vi "Destroy.vi"   [LabVIEW 2018, in "Toolkit.lvlib" / "Channel.lvclass"]
uses:
  Channel.lvclass
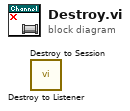
[diagram p0: block diagram]
diagram:
  n1 = call "Destroy to Listener.vi"() -> ()  [unwired: 10 in, 2 out]
  n2 = call "Destroy to Session.vi"() -> ()  [unwired: 10 in, 2 out]
